vi "S4GUI_002.vi"(7 "Tab ObsEng":enum32{"Obs", "CCD modes", "Eng"}(tab)) -> ()   [LabVIEW 2018] (continued)
            n3730 = call-dynamic "Write Observer.vi"("error in (no error)"=w8546, "Observer"=w8544, "Interface in"=w8548) -> ("error out"=w8545:errorcluster, "Interface out"=w8547:refnum<class "Interface.lvclass">)  [unwired: 7 in]
            n3731 = call-dynamic "Write # Images.vi"("error in (no error)"=w8545, "# Images"="Exp ch4", "Interface in"=w8547) -> ("error out"=w8551:errorcluster, "Interface out"=w8552:refnum<class "Interface.lvclass">)  [unwired: 7 in]
            n3732 = property on="Exposure Time ch4" class="Slide (strict)"("Scale.Maximum"="Exptime ch4", "Scale.Minimum"=0.0 ("Scale.Range:Minimum")) -> ()  [unwired: 2 in, 2 out]
            n3733 = property on="Exposures Done ch4" class="Slide (strict)"("Scale.Maximum"="Exp ch4", "Scale.Minimum"=0.0 ("Scale.Range:Minimum")) -> ()  [unwired: 2 in, 2 out]
            n3734 = call-dynamic "Write Interface.vi"("error in (no error)"=w8551, "Interface.lvclass"=w8552, "Channel in"=w8579) -> ("error out"=w8561:errorcluster, "Channel out"=w8562:refnum<class "Channel.lvclass">)  [unwired: 7 in]
            n3735 = property on="Cycles Done ch4" class="Slide (strict)"("Scale.Maximum"=w8533, "Scale.Minimum"=0.0 ("Scale.Range:Minimum")) -> ()  [unwired: 2 in, 2 out]
            n3736 = call-dynamic "Write ciclos.vi"("error in (no error)"=w8561, "ciclos"=w8533, "Channel in"=w8562) -> ("error out"=w8542:errorcluster, "Channel out"=w8543:refnum<class "Channel.lvclass">)  [unwired: 7 in]
            n3737 = call-dynamic "Write sequencias.vi"("error in (no error)"=w8542, "sequencias"=w8531, "Channel in"=w8543) -> ("error out"=w8541:errorcluster, "Channel out"=w8540:refnum<class "Channel.lvclass">)  [unwired: 7 in]
            n3738 = call-dynamic "Write Channel.vi"("error in (no error)"=w8541, "Channel.lvclass"=w8540, "Acquisition in"=w8568) -> ("error out"=w8508:errorcluster, "Acquisition out"=w8509:refnum<class "Acquisition.lvclass">)  [unwired: 7 in]
            n3739 = call-dynamic "CalcCubeDuration.vi"("error in (no error)"=w8508, "Acquisition in"=w8509) -> ("error out"=w8507:errorcluster, "Acquisition out"=w8506:refnum<class "Acquisition.lvclass">)  [unwired: 8 in]
            n3740 = call-dynamic "Write sequencias.vi"("error in (no error)"=w8507, "sequencias"=w8531, "S4GUI in"=w8514) -> ("error out"=w8537:errorcluster, "S4GUI out"=w8536:refnum<class "S4GUI.lvclass">)  [unwired: 7 in]
            n3741 = call-dynamic "Write ciclos.vi"("error in (no error)"=w8537, "ciclos"=w8533, "S4ACS_GUI in"=w8536) -> ("error out"=w8538:errorcluster, "S4ACS_GUI out"=w8539:refnum<class "S4GUI.lvclass">)  [unwired: 7 in]
            n3742 = call-dynamic "Write TotalCiclos.vi"("error in (no error)"=w8538, "TotalCiclos"=w8533, "S4GUI in"=w8539) -> ("error out"=w8534:errorcluster, "S4GUI out"=w8535:refnum<class "S4GUI.lvclass">)  [unwired: 7 in]
          }
        }
        n3743 = call-dynamic "Write AcquisitionD.vi"("error in (no error)"=w8452, "Acquisition.lvclass"=w8467, "S4ACS_GUI in"=w8451) -> ("error out"=w8466:errorcluster, "S4ACS_GUI out"=w8463:refnum<class "S4GUI.lvclass">)  [unwired: 7 in]
      }
      event "Exptime ch1": Value Change {
        n3744 = event-data() -> ("NewVal"=w8618:dbl)  [unwired: 1 in]
        n3745 = call-dynamic "Read AcquisitionA.vi"("error in (no error)"=w8617, "S4ACS_GUI in"=w8616) -> ("error out"=w8632:errorcluster, "Acquisition.lvclass"=w8633:refnum<class "Acquisition.lvclass">, "S4ACS_GUI out"=w8630:refnum<class "S4GUI.lvclass">)  [unwired: 7 in]
        n3746 = call-dynamic "Read Channel.vi"("error in (no error)"=w8632, "Acquisition in"=w8633) -> ("error out"=w8621:errorcluster, "Channel.lvclass"=w8622:refnum<class "Channel.lvclass">, "Acquisition out"=w8623:refnum<class "Acquisition.lvclass">)  [unwired: 7 in]
        n3747 = call-dynamic "Read Interface.vi"("error in (no error)"=w8621, "Channel in"=w8622) -> ("error out"=w8627:errorcluster, "Interface.lvclass"=w8628:refnum<class "Interface.lvclass">, "Channel out"=w8626:refnum<class "Channel.lvclass">)  [unwired: 7 in]
        n3748 = call "Write Exposure Time.vi"("error in (no error)"=w8627, "Exposure Time"=w8618, "Interface in"=w8628) -> ("error out"=w8619:errorcluster, "Interface out"=w8620:refnum<class "Interface.lvclass">)  [unwired: 7 in]
        n3749 = call-dynamic "Write Interface.vi"("error in (no error)"=w8619, "Interface.lvclass"=w8620, "Channel in"=w8626) -> ("error out"=w8625:errorcluster, "Channel out"=w8624:refnum<class "Channel.lvclass">)  [unwired: 7 in]
        n3750 = call-dynamic "Write Channel.vi"("error in (no error)"=w8625, "Channel.lvclass"=w8624, "Acquisition in"=w8623) -> ("error out"=w8629:errorcluster, "Acquisition out"=w8631:refnum<class "Acquisition.lvclass">)  [unwired: 7 in]
        n3751 = call-dynamic "Write AcquisitionA.vi"("error in (no error)"=w8629, "Acquisition.lvclass"=w8631, "S4ACS_GUI in"=w8630) -> ("error out"=w8615:errorcluster, "S4ACS_GUI out"=w8614:refnum<class "S4GUI.lvclass">)  [unwired: 7 in]
      }
      event "Exptime ch2": Value Change {
        n3752 = event-data() -> ("NewVal"=w8638:dbl)  [unwired: 1 in]
        n3753 = call "Read AcquisitionB.vi"("error in (no error)"=w8637, "S4ACS_GUI in"=w8636) -> ("error out"=w8652:errorcluster, "Acquisition.lvclass"=w8653:refnum<class "Acquisition.lvclass">, "S4ACS_GUI out"=w8650:refnum<class "S4GUI.lvclass">)  [unwired: 7 in]
        n3754 = call-dynamic "Read Channel.vi"("error in (no error)"=w8652, "Acquisition in"=w8653) -> ("error out"=w8641:errorcluster, "Channel.lvclass"=w8642:refnum<class "Channel.lvclass">, "Acquisition out"=w8643:refnum<class "Acquisition.lvclass">)  [unwired: 7 in]
        n3755 = call-dynamic "Read Interface.vi"("error in (no error)"=w8641, "Channel in"=w8642) -> ("error out"=w8647:errorcluster, "Interface.lvclass"=w8648:refnum<class "Interface.lvclass">, "Channel out"=w8646:refnum<class "Channel.lvclass">)  [unwired: 7 in]
        n3756 = call "Write Exposure Time.vi"("error in (no error)"=w8647, "Exposure Time"=w8638, "Interface in"=w8648) -> ("error out"=w8639:errorcluster, "Interface out"=w8640:refnum<class "Interface.lvclass">)  [unwired: 7 in]
        n3757 = call-dynamic "Write Interface.vi"("error in (no error)"=w8639, "Interface.lvclass"=w8640, "Channel in"=w8646) -> ("error out"=w8645:errorcluster, "Channel out"=w8644:refnum<class "Channel.lvclass">)  [unwired: 7 in]
        n3758 = call-dynamic "Write Channel.vi"("error in (no error)"=w8645, "Channel.lvclass"=w8644, "Acquisition in"=w8643) -> ("error out"=w8649:errorcluster, "Acquisition out"=w8651:refnum<class "Acquisition.lvclass">)  [unwired: 7 in]
        n3759 = call "Write AcquisitionB.vi"("error in (no error)"=w8649, "Acquisition.lvclass"=w8651, "S4ACS_GUI in"=w8650) -> ("error out"=w8635:errorcluster, "S4ACS_GUI out"=w8634:refnum<class "S4GUI.lvclass">)  [unwired: 7 in]
      }
      event "Exptime ch3": Value Change {
        n3760 = event-data() -> ("NewVal"=w8658:dbl)  [unwired: 1 in]
        n3761 = call-dynamic "Read AcquisitionC.vi"("error in (no error)"=w8657, "S4ACS_GUI in"=w8656) -> ("error out"=w8672:errorcluster, "Acquisition.lvclass"=w8673:refnum<class "Acquisition.lvclass">, "S4ACS_GUI out"=w8670:refnum<class "S4GUI.lvclass">)  [unwired: 7 in]
        n3762 = call-dynamic "Read Channel.vi"("error in (no error)"=w8672, "Acquisition in"=w8673) -> ("error out"=w8661:errorcluster, "Channel.lvclass"=w8662:refnum<class "Channel.lvclass">, "Acquisition out"=w8663:refnum<class "Acquisition.lvclass">)  [unwired: 7 in]
        n3763 = call-dynamic "Read Interface.vi"("error in (no error)"=w8661, "Channel in"=w8662) -> ("error out"=w8667:errorcluster, "Interface.lvclass"=w8668:refnum<class "Interface.lvclass">, "Channel out"=w8666:refnum<class "Channel.lvclass">)  [unwired: 7 in]
        n3764 = call "Write Exposure Time.vi"("error in (no error)"=w8667, "Exposure Time"=w8658, "Interface in"=w8668) -> ("error out"=w8659:errorcluster, "Interface out"=w8660:refnum<class "Interface.lvclass">)  [unwired: 7 in]
        n3765 = call-dynamic "Write Interface.vi"("error in (no error)"=w8659, "Interface.lvclass"=w8660, "Channel in"=w8666) -> ("error out"=w8665:errorcluster, "Channel out"=w8664:refnum<class "Channel.lvclass">)  [unwired: 7 in]
        n3766 = call-dynamic "Write Channel.vi"("error in (no error)"=w8665, "Channel.lvclass"=w8664, "Acquisition in"=w8663) -> ("error out"=w8669:errorcluster, "Acquisition out"=w8671:refnum<class "Acquisition.lvclass">)  [unwired: 7 in]
        n3767 = call-dynamic "Write AcquisitionC.vi"("error in (no error)"=w8669, "Acquisition.lvclass"=w8671, "S4ACS_GUI in"=w8670) -> ("error out"=w8655:errorcluster, "S4ACS_GUI out"=w8654:refnum<class "S4GUI.lvclass">)  [unwired: 7 in]
      }
      event "Exptime ch4": Value Change {
        n3768 = event-data() -> ("NewVal"=w8678:dbl)  [unwired: 1 in]
        n3769 = call-dynamic "Read AcquisitionD.vi"("error in (no error)"=w8677, "S4ACS_GUI in"=w8676) -> ("error out"=w8692:errorcluster, "Acquisition.lvclass"=w8693:refnum<class "Acquisition.lvclass">, "S4ACS_GUI out"=w8690:refnum<class "S4GUI.lvclass">)  [unwired: 7 in]
        n3770 = call-dynamic "Read Channel.vi"("error in (no error)"=w8692, "Acquisition in"=w8693) -> ("error out"=w8681:errorcluster, "Channel.lvclass"=w8682:refnum<class "Channel.lvclass">, "Acquisition out"=w8683:refnum<class "Acquisition.lvclass">)  [unwired: 7 in]
        n3771 = call-dynamic "Read Interface.vi"("error in (no error)"=w8681, "Channel in"=w8682) -> ("error out"=w8687:errorcluster, "Interface.lvclass"=w8688:refnum<class "Interface.lvclass">, "Channel out"=w8686:refnum<class "Channel.lvclass">)  [unwired: 7 in]
        n3772 = call "Write Exposure Time.vi"("error in (no error)"=w8687, "Exposure Time"=w8678, "Interface in"=w8688) -> ("error out"=w8679:errorcluster, "Interface out"=w8680:refnum<class "Interface.lvclass">)  [unwired: 7 in]
        n3773 = call-dynamic "Write Interface.vi"("error in (no error)"=w8679, "Interface.lvclass"=w8680, "Channel in"=w8686) -> ("error out"=w8685:errorcluster, "Channel out"=w8684:refnum<class "Channel.lvclass">)  [unwired: 7 in]
        n3774 = call-dynamic "Write Channel.vi"("error in (no error)"=w8685, "Channel.lvclass"=w8684, "Acquisition in"=w8683) -> ("error out"=w8689:errorcluster, "Acquisition out"=w8691:refnum<class "Acquisition.lvclass">)  [unwired: 7 in]
        n3775 = call-dynamic "Write AcquisitionD.vi"("error in (no error)"=w8689, "Acquisition.lvclass"=w8691, "S4ACS_GUI in"=w8690) -> ("error out"=w8675:errorcluster, "S4ACS_GUI out"=w8674:refnum<class "S4GUI.lvclass">)  [unwired: 7 in]
      }
      event "Stop ch1": Value Change {
        n3776 = event-data() -> ()  [unwired: 1 in, 6 out]
        n3777 = disable-structure shown="Enabled" {
          disable-tunnel: w8697 -> [w8730 w8758]
          disable-tunnel: w8696 -> [w8728 w8752]
          disable-tunnel: [w8710 w8751] -> w8695
          disable-tunnel: [w8698 w8758] -> w8694
          frame Disabled {
            # "Para movimento \nda lamina retardadora"
            # "Restaura a última sequência de lâminas"
            n3778 = call-dynamic "Read AcquisitionA.vi"("error in (no error)"=w8728, "S4ACS_GUI in"=w8730) -> ("error out"=w8732:errorcluster, "Acquisition.lvclass"=w8731:refnum<class "Acquisition.lvclass">, "S4ACS_GUI out"=w8729:refnum<class "S4GUI.lvclass">)  [unwired: 7 in]
            n3779 = disable-structure shown="Enabled" {
              disable-tunnel: w8732 -> [w8737 w8748]
              disable-tunnel: w8731 -> [w8736 w8749]
              disable-tunnel: [w8734 w8749] -> w8726
              disable-tunnel: [w8733 w8748] -> w8725
              frame Disabled {
                # "Só precisa enviar comando STOP quando\no controle dos ciclos for feito pelo ACS."
                n3780 = call-dynamic "Read Channel.vi"("error in (no error)"=w8737, "Acquisition in"=w8736) -> ("error out"=w8739:errorcluster, "Channel.lvclass"=w8738:refnum<class "Channel.lvclass">, "Acquisition out"=w8745:refnum<class "Acquisition.lvclass">)  [unwired: 7 in]
                n3781 = call-dynamic "Read State Machine.vi"("error in (no error)"=w8739, "Device in"=w8738) -> ("error out"=w8741:errorcluster, "State Machine.lvclass"=w8740:refnum<class "State Machine.lvclass">, "Device out"=w8743:refnum<class "Channel.lvclass">)  [unwired: 7 in]
                n3782 = call "Next State.vi"("error in (no error)"=w8741, "New_State"=u32 70, "State Machine in"=w8740) -> ("error out"=w8744:errorcluster, "State Machine out"=w8742:refnum<class "State Machine.lvclass">)  [unwired: 7 in]
                n3783 = call-dynamic "Write State Machine.vi"("error in (no error)"=w8744, "State Machine.lvclass"=w8742, "Device in"=w8743) -> ("error out"=w8746:errorcluster, "Device out"=w8747:refnum<class "Channel.lvclass">)  [unwired: 7 in]
                n3784 = call-dynamic "Write Channel.vi"("error in (no error)"=w8746, "Channel.lvclass"=w8747, "Acquisition in"=w8745) -> ("error out"=w8733:errorcluster, "Acquisition out"=w8734:refnum<class "Acquisition.lvclass">)  [unwired: 7 in]
              }
              frame Enabled {
                # "Não precisa enviar comando STOP para o ACS\nenquanto o controle dos ciclos for feito pela GUI."
              }
            }
            n3785 = call-dynamic "Write Acq_state.vi"("error in (no error)"=w8725, "Acq_state"=u32 0, "Acquisition in"=w8726) -> ("error out"=w8724:errorcluster, "Acquisition out"=w8723:refnum<class "Acquisition.lvclass">)  [unwired: 7 in]
            n3786 = call-dynamic "Write AcquisitionA.vi"("error in (no error)"=w8724, "Acquisition.lvclass"=w8723, "S4ACS_GUI in"=w8729) -> ("error out"=w8711:errorcluster, "S4ACS_GUI out"=w8709:refnum<class "S4GUI.lvclass">)  [unwired: 7 in]
            n3787 = call "Read Instrument.lvclass.vi"("error in (no error)"=w8711, "S4ACS_GUI in"=w8709) -> ("error out"=w8718:errorcluster, "Instrument.lvclass"=w8721:refnum<class "Instrument.lvclass">, "S4ACS_GUI out"=w8722:refnum<class "S4GUI.lvclass">)  [unwired: 7 in]
            n3788 = call "Read WPROT.vi"("error in (no error)"=w8718, "Instrument in"=w8721) -> ("error out"=w8717:errorcluster, "Opt_Selector.lvclass"=w8719:refnum<class "Opt_Selector.lvclass">, "Instrument out"=w8720:refnum<class "Instrument.lvclass">)  [unwired: 7 in]
            n3789 = call-dynamic "Read sequencia_ant.vi"("error in (no error)"=w8717, "Opt_Selector in"=w8719) -> ("error out"=w8713:errorcluster, "sequencia_ant"=w8712:u16, "Opt_Selector out"=w8714:refnum<class "Opt_Selector.lvclass">)  [unwired: 7 in]
            n3790 = call-dynamic "Write sequencia.vi"("error in (no error)"=w8713, "sequencia"=w8712, "Opt_Selector in"=w8714) -> ("error out"=w8700:errorcluster, "Opt_Selector out"=w8703:refnum<class "Opt_Selector.lvclass">)  [unwired: 7 in]
            n3791 = call-dynamic "Read State Machine.vi"("error in (no error)"=w8700, "Device in"=w8703) -> ("error out"=w8705:errorcluster, "State Machine.lvclass"=w8708:refnum<class "State Machine.lvclass">, "Device out"=w8702:refnum<class "Opt_Selector.lvclass">)  [unwired: 7 in]
            n3792 = call "Next State.vi"("error in (no error)"=w8705, "New_State"=10, "State Machine in"=w8708) -> ("error out"=w8704:errorcluster, "State Machine out"=w8707:refnum<class "State Machine.lvclass">)  [unwired: 7 in]
            n3793 = call-dynamic "Write State Machine.vi"("error in (no error)"=w8704, "State Machine.lvclass"=w8707, "Device in"=w8702) -> ("error out"=w8699:errorcluster, "Device out"=w8701:refnum<class "Opt_Selector.lvclass">)  [unwired: 7 in]
            n3794 = call "Write WPROT.vi"("error in (no error)"=w8699, "Opt_Selector.lvclass"=w8701, "Instrument in"=w8720) -> ("error out"=w8716:errorcluster, "Instrument out"=w8715:refnum<class "Instrument.lvclass">)  [unwired: 7 in]
            n3795 = call "Write Instrument.lvclass.vi"("error in (no error)"=w8716, "Instrument.lvclass"=w8715, "S4ACS_GUI in"=w8722) -> ("error out"=w8710:errorcluster, "S4ACS_GUI out"=w8698:refnum<class "S4GUI.lvclass">)  [unwired: 7 in]
          }
          frame Enabled {
            w8754 = FALSE ("Wait Until Done")
            n3796 = call <vilib>:"Application Directory.vi"() -> ("Application Directory"=w8750:path)
            n3797 = Build Path(base path=w8750, name or relative path="MsgStop1.vi") -> (appended path=w8757:path)
            n3798 = Open VI Reference(vi path=w8757, error in (no error)=w8752) -> (vi reference=w8756:refnum<vi>, error out=w8755:errorcluster)  [unwired: 4 in]
            n3799 = invoke class="VI" method="Run VI"(reference=w8756, error in=w8755, "Wait until done"=w8754, "Auto Dispose Ref"=w8754) -> (error out=w8751:errorcluster)  [unwired: 1 in, 4 out]
          }
        }
      }
      event "Stop ch2": Value Change {
        n3800 = event-data() -> ()  [unwired: 1 in, 6 out]
        n3801 = disable-structure shown="Enabled" {
          disable-tunnel: w8762 -> [w8795 w8816]
          disable-tunnel: w8761 -> [w8793 w8818]
          disable-tunnel: [w8775 w8817] -> w8760
          disable-tunnel: [w8763 w8816] -> w8759
          frame Disabled {
            # "Para movimento \nda lamina retardadora"
            # "Restaura a última sequência de lâminas"
            n3802 = call "Read AcquisitionB.vi"("error in (no error)"=w8793, "S4ACS_GUI in"=w8795) -> ("error out"=w8797:errorcluster, "Acquisition.lvclass"=w8796:refnum<class "Acquisition.lvclass">, "S4ACS_GUI out"=w8794:refnum<class "S4GUI.lvclass">)  [unwired: 7 in]
            n3803 = disable-structure shown="Enabled" {
              disable-tunnel: w8797 -> [w8802 w8813]
              disable-tunnel: w8796 -> [w8801 w8814]
              disable-tunnel: [w8799 w8814] -> w8791
              disable-tunnel: [w8798 w8813] -> w8790
              frame Disabled {
                # "Só precisa enviar comando STOP quando\no controle dos ciclos for feito pelo ACS."
                n3804 = call-dynamic "Read Channel.vi"("error in (no error)"=w8802, "Acquisition in"=w8801) -> ("error out"=w8804:errorcluster, "Channel.lvclass"=w8803:refnum<class "Channel.lvclass">, "Acquisition out"=w8810:refnum<class "Acquisition.lvclass">)  [unwired: 7 in]
                n3805 = call-dynamic "Read State Machine.vi"("error in (no error)"=w8804, "Device in"=w8803) -> ("error out"=w8806:errorcluster, "State Machine.lvclass"=w8805:refnum<class "State Machine.lvclass">, "Device out"=w8808:refnum<class "Channel.lvclass">)  [unwired: 7 in]
                n3806 = call "Next State.vi"("error in (no error)"=w8806, "New_State"=u32 70, "State Machine in"=w8805) -> ("error out"=w8809:errorcluster, "State Machine out"=w8807:refnum<class "State Machine.lvclass">)  [unwired: 7 in]
                n3807 = call-dynamic "Write State Machine.vi"("error in (no error)"=w8809, "State Machine.lvclass"=w8807, "Device in"=w8808) -> ("error out"=w8811:errorcluster, "Device out"=w8812:refnum<class "Channel.lvclass">)  [unwired: 7 in]
                n3808 = call-dynamic "Write Channel.vi"("error in (no error)"=w8811, "Channel.lvclass"=w8812, "Acquisition in"=w8810) -> ("error out"=w8798:errorcluster, "Acquisition out"=w8799:refnum<class "Acquisition.lvclass">)  [unwired: 7 in]
              }
              frame Enabled {
                # "Não precisa enviar comando STOP para o ACS\nenquanto o controle dos ciclos for feito pela GUI."
              }
            }
            n3809 = call-dynamic "Write Acq_state.vi"("error in (no error)"=w8790, "Acq_state"=u32 0, "Acquisition in"=w8791) -> ("error out"=w8789:errorcluster, "Acquisition out"=w8788:refnum<class "Acquisition.lvclass">)  [unwired: 7 in]
            n3810 = call "Write AcquisitionB.vi"("error in (no error)"=w8789, "Acquisition.lvclass"=w8788, "S4ACS_GUI in"=w8794) -> ("error out"=w8776:errorcluster, "S4ACS_GUI out"=w8774:refnum<class "S4GUI.lvclass">)  [unwired: 7 in]
            n3811 = call "Read Instrument.lvclass.vi"("error in (no error)"=w8776, "S4ACS_GUI in"=w8774) -> ("error out"=w8783:errorcluster, "Instrument.lvclass"=w8786:refnum<class "Instrument.lvclass">, "S4ACS_GUI out"=w8787:refnum<class "S4GUI.lvclass">)  [unwired: 7 in]
            n3812 = call "Read WPROT.vi"("error in (no error)"=w8783, "Instrument in"=w8786) -> ("error out"=w8782:errorcluster, "Opt_Selector.lvclass"=w8784:refnum<class "Opt_Selector.lvclass">, "Instrument out"=w8785:refnum<class "Instrument.lvclass">)  [unwired: 7 in]
            n3813 = call-dynamic "Read sequencia_ant.vi"("error in (no error)"=w8782, "Opt_Selector in"=w8784) -> ("error out"=w8778:errorcluster, "sequencia_ant"=w8777:u16, "Opt_Selector out"=w8779:refnum<class "Opt_Selector.lvclass">)  [unwired: 7 in]
            n3814 = call-dynamic "Write sequencia.vi"("error in (no error)"=w8778, "sequencia"=w8777, "Opt_Selector in"=w8779) -> ("error out"=w8765:errorcluster, "Opt_Selector out"=w8768:refnum<class "Opt_Selector.lvclass">)  [unwired: 7 in]
            n3815 = call-dynamic "Read State Machine.vi"("error in (no error)"=w8765, "Device in"=w8768) -> ("error out"=w8770:errorcluster, "State Machine.lvclass"=w8773:refnum<class "State Machine.lvclass">, "Device out"=w8767:refnum<class "Opt_Selector.lvclass">)  [unwired: 7 in]
            n3816 = call "Next State.vi"("error in (no error)"=w8770, "New_State"=10, "State Machine in"=w8773) -> ("error out"=w8769:errorcluster, "State Machine out"=w8772:refnum<class "State Machine.lvclass">)  [unwired: 7 in]
            n3817 = call-dynamic "Write State Machine.vi"("error in (no error)"=w8769, "State Machine.lvclass"=w8772, "Device in"=w8767) -> ("error out"=w8764:errorcluster, "Device out"=w8766:refnum<class "Opt_Selector.lvclass">)  [unwired: 7 in]
            n3818 = call "Write WPROT.vi"("error in (no error)"=w8764, "Opt_Selector.lvclass"=w8766, "Instrument in"=w8785) -> ("error out"=w8781:errorcluster, "Instrument out"=w8780:refnum<class "Instrument.lvclass">)  [unwired: 7 in]
            n3819 = call "Write Instrument.lvclass.vi"("error in (no error)"=w8781, "Instrument.lvclass"=w8780, "S4ACS_GUI in"=w8787) -> ("error out"=w8775:errorcluster, "S4ACS_GUI out"=w8763:refnum<class "S4GUI.lvclass">)  [unwired: 7 in]
          }
          frame Enabled {
            w8820 = FALSE ("Wait Until Done")
            n3820 = call <vilib>:"Application Directory.vi"() -> ("Application Directory"=w8815:path)
            n3821 = Build Path(base path=w8815, name or relative path="MsgStop2.vi") -> (appended path=w8823:path)
            n3822 = Open VI Reference(vi path=w8823, error in (no error)=w8818) -> (vi reference=w8822:refnum<vi>, error out=w8821:errorcluster)  [unwired: 4 in]
            n3823 = invoke class="VI" method="Run VI"(reference=w8822, error in=w8821, "Wait until done"=w8820, "Auto Dispose Ref"=w8820) -> (error out=w8817:errorcluster)  [unwired: 1 in, 4 out]
          }
        }
      }
      event "Stop ch3": Value Change {
        n3824 = event-data() -> ()  [unwired: 1 in, 6 out]
        n3825 = disable-structure shown="Enabled" {
          disable-tunnel: w8827 -> [w8860 w8881]
          disable-tunnel: w8826 -> [w8858 w8883]
          disable-tunnel: [w8840 w8882] -> w8825
          disable-tunnel: [w8828 w8881] -> w8824
          frame Disabled {
            # "Para movimento \nda lamina retardadora"
            # "Restaura a última sequência de lâminas"
            n3826 = call-dynamic "Read AcquisitionC.vi"("error in (no error)"=w8858, "S4ACS_GUI in"=w8860) -> ("error out"=w8862:errorcluster, "Acquisition.lvclass"=w8861:refnum<class "Acquisition.lvclass">, "S4ACS_GUI out"=w8859:refnum<class "S4GUI.lvclass">)  [unwired: 7 in]
            n3827 = disable-structure shown="Enabled" {
              disable-tunnel: w8862 -> [w8867 w8878]
              disable-tunnel: w8861 -> [w8866 w8879]
              disable-tunnel: [w8864 w8879] -> w8856
              disable-tunnel: [w8863 w8878] -> w8855
              frame Disabled {
                # "Só precisa enviar comando STOP quando\no controle dos ciclos for feito pelo ACS."
                n3828 = call-dynamic "Read Channel.vi"("error in (no error)"=w8867, "Acquisition in"=w8866) -> ("error out"=w8869:errorcluster, "Channel.lvclass"=w8868:refnum<class "Channel.lvclass">, "Acquisition out"=w8875:refnum<class "Acquisition.lvclass">)  [unwired: 7 in]
                n3829 = call-dynamic "Read State Machine.vi"("error in (no error)"=w8869, "Device in"=w8868) -> ("error out"=w8871:errorcluster, "State Machine.lvclass"=w8870:refnum<class "State Machine.lvclass">, "Device out"=w8873:refnum<class "Channel.lvclass">)  [unwired: 7 in]
                n3830 = call "Next State.vi"("error in (no error)"=w8871, "New_State"=u32 70, "State Machine in"=w8870) -> ("error out"=w8874:errorcluster, "State Machine out"=w8872:refnum<class "State Machine.lvclass">)  [unwired: 7 in]
                n3831 = call-dynamic "Write State Machine.vi"("error in (no error)"=w8874, "State Machine.lvclass"=w8872, "Device in"=w8873) -> ("error out"=w8876:errorcluster, "Device out"=w8877:refnum<class "Channel.lvclass">)  [unwired: 7 in]
                n3832 = call-dynamic "Write Channel.vi"("error in (no error)"=w8876, "Channel.lvclass"=w8877, "Acquisition in"=w8875) -> ("error out"=w8863:errorcluster, "Acquisition out"=w8864:refnum<class "Acquisition.lvclass">)  [unwired: 7 in]
              }
              frame Enabled {
                # "Não precisa enviar comando STOP para o ACS\nenquanto o controle dos ciclos for feito pela GUI."
              }
            }
            n3833 = call-dynamic "Write Acq_state.vi"("error in (no error)"=w8855, "Acq_state"=u32 0, "Acquisition in"=w8856) -> ("error out"=w8854:errorcluster, "Acquisition out"=w8853:refnum<class "Acquisition.lvclass">)  [unwired: 7 in]
            n3834 = call-dynamic "Write AcquisitionC.vi"("error in (no error)"=w8854, "Acquisition.lvclass"=w8853, "S4ACS_GUI in"=w8859) -> ("error out"=w8841:errorcluster, "S4ACS_GUI out"=w8839:refnum<class "S4GUI.lvclass">)  [unwired: 7 in]
            n3835 = call "Read Instrument.lvclass.vi"("error in (no error)"=w8841, "S4ACS_GUI in"=w8839) -> ("error out"=w8848:errorcluster, "Instrument.lvclass"=w8851:refnum<class "Instrument.lvclass">, "S4ACS_GUI out"=w8852:refnum<class "S4GUI.lvclass">)  [unwired: 7 in]
            n3836 = call "Read WPROT.vi"("error in (no error)"=w8848, "Instrument in"=w8851) -> ("error out"=w8847:errorcluster, "Opt_Selector.lvclass"=w8849:refnum<class "Opt_Selector.lvclass">, "Instrument out"=w8850:refnum<class "Instrument.lvclass">)  [unwired: 7 in]
            n3837 = call-dynamic "Read sequencia_ant.vi"("error in (no error)"=w8847, "Opt_Selector in"=w8849) -> ("error out"=w8843:errorcluster, "sequencia_ant"=w8842:u16, "Opt_Selector out"=w8844:refnum<class "Opt_Selector.lvclass">)  [unwired: 7 in]
            n3838 = call-dynamic "Write sequencia.vi"("error in (no error)"=w8843, "sequencia"=w8842, "Opt_Selector in"=w8844) -> ("error out"=w8830:errorcluster, "Opt_Selector out"=w8833:refnum<class "Opt_Selector.lvclass">)  [unwired: 7 in]
            n3839 = call-dynamic "Read State Machine.vi"("error in (no error)"=w8830, "Device in"=w8833) -> ("error out"=w8835:errorcluster, "State Machine.lvclass"=w8838:refnum<class "State Machine.lvclass">, "Device out"=w8832:refnum<class "Opt_Selector.lvclass">)  [unwired: 7 in]
            n3840 = call "Next State.vi"("error in (no error)"=w8835, "New_State"=10, "State Machine in"=w8838) -> ("error out"=w8834:errorcluster, "State Machine out"=w8837:refnum<class "State Machine.lvclass">)  [unwired: 7 in]
            n3841 = call-dynamic "Write State Machine.vi"("error in (no error)"=w8834, "State Machine.lvclass"=w8837, "Device in"=w8832) -> ("error out"=w8829:errorcluster, "Device out"=w8831:refnum<class "Opt_Selector.lvclass">)  [unwired: 7 in]
            n3842 = call "Write WPROT.vi"("error in (no error)"=w8829, "Opt_Selector.lvclass"=w8831, "Instrument in"=w8850) -> ("error out"=w8846:errorcluster, "Instrument out"=w8845:refnum<class "Instrument.lvclass">)  [unwired: 7 in]
            n3843 = call "Write Instrument.lvclass.vi"("error in (no error)"=w8846, "Instrument.lvclass"=w8845, "S4ACS_GUI in"=w8852) -> ("error out"=w8840:errorcluster, "S4ACS_GUI out"=w8828:refnum<class "S4GUI.lvclass">)  [unwired: 7 in]
          }
          frame Enabled {
            w8885 = FALSE ("Wait Until Done")
            n3844 = call <vilib>:"Application Directory.vi"() -> ("Application Directory"=w8880:path)
            n3845 = Build Path(base path=w8880, name or relative path="MsgStop3.vi") -> (appended path=w8888:path)
            n3846 = Open VI Reference(vi path=w8888, error in (no error)=w8883) -> (vi reference=w8887:refnum<vi>, error out=w8886:errorcluster)  [unwired: 4 in]
            n3847 = invoke class="VI" method="Run VI"(reference=w8887, error in=w8886, "Wait until done"=w8885, "Auto Dispose Ref"=w8885) -> (error out=w8882:errorcluster)  [unwired: 1 in, 4 out]
          }
        }
      }
      event "Stop ch4": Value Change {
        n3848 = event-data() -> ()  [unwired: 1 in, 6 out]
        n3849 = disable-structure shown="Enabled" {
          disable-tunnel: w8892 -> [w8925 w8946]
          disable-tunnel: w8891 -> [w8923 w8948]
          disable-tunnel: [w8905 w8947] -> w8890
          disable-tunnel: [w8893 w8946] -> w8889
          frame Disabled {
            # "Para movimento \nda lamina retardadora"
            # "Restaura a última sequência de lâminas"
            n3850 = call-dynamic "Read AcquisitionD.vi"("error in (no error)"=w8923, "S4ACS_GUI in"=w8925) -> ("error out"=w8927:errorcluster, "Acquisition.lvclass"=w8926:refnum<class "Acquisition.lvclass">, "S4ACS_GUI out"=w8924:refnum<class "S4GUI.lvclass">)  [unwired: 7 in]
            n3851 = disable-structure shown="Enabled" {
              disable-tunnel: w8927 -> [w8932 w8943]
              disable-tunnel: w8926 -> [w8931 w8944]
              disable-tunnel: [w8929 w8944] -> w8921
              disable-tunnel: [w8928 w8943] -> w8920
              frame Disabled {
                # "Só precisa enviar comando STOP quando\no controle dos ciclos for feito pelo ACS."
                n3852 = call-dynamic "Read Channel.vi"("error in (no error)"=w8932, "Acquisition in"=w8931) -> ("error out"=w8934:errorcluster, "Channel.lvclass"=w8933:refnum<class "Channel.lvclass">, "Acquisition out"=w8940:refnum<class "Acquisition.lvclass">)  [unwired: 7 in]
                n3853 = call-dynamic "Read State Machine.vi"("error in (no error)"=w8934, "Device in"=w8933) -> ("error out"=w8936:errorcluster, "State Machine.lvclass"=w8935:refnum<class "State Machine.lvclass">, "Device out"=w8938:refnum<class "Channel.lvclass">)  [unwired: 7 in]
                n3854 = call "Next State.vi"("error in (no error)"=w8936, "New_State"=u32 70, "State Machine in"=w8935) -> ("error out"=w8939:errorcluster, "State Machine out"=w8937:refnum<class "State Machine.lvclass">)  [unwired: 7 in]
                n3855 = call-dynamic "Write State Machine.vi"("error in (no error)"=w8939, "State Machine.lvclass"=w8937, "Device in"=w8938) -> ("error out"=w8941:errorcluster, "Device out"=w8942:refnum<class "Channel.lvclass">)  [unwired: 7 in]
                n3856 = call-dynamic "Write Channel.vi"("error in (no error)"=w8941, "Channel.lvclass"=w8942, "Acquisition in"=w8940) -> ("error out"=w8928:errorcluster, "Acquisition out"=w8929:refnum<class "Acquisition.lvclass">)  [unwired: 7 in]
              }
              frame Enabled {
                # "Não precisa enviar comando STOP para o ACS\nenquanto o controle dos ciclos for feito pela GUI."
              }
            }
            n3857 = call-dynamic "Write Acq_state.vi"("error in (no error)"=w8920, "Acq_state"=u32 0, "Acquisition in"=w8921) -> ("error out"=w8919:errorcluster, "Acquisition out"=w8918:refnum<class "Acquisition.lvclass">)  [unwired: 7 in]
            n3858 = call-dynamic "Write AcquisitionD.vi"("error in (no error)"=w8919, "Acquisition.lvclass"=w8918, "S4ACS_GUI in"=w8924) -> ("error out"=w8906:errorcluster, "S4ACS_GUI out"=w8904:refnum<class "S4GUI.lvclass">)  [unwired: 7 in]
            n3859 = call "Read Instrument.lvclass.vi"("error in (no error)"=w8906, "S4ACS_GUI in"=w8904) -> ("error out"=w8913:errorcluster, "Instrument.lvclass"=w8916:refnum<class "Instrument.lvclass">, "S4ACS_GUI out"=w8917:refnum<class "S4GUI.lvclass">)  [unwired: 7 in]
            n3860 = call "Read WPROT.vi"("error in (no error)"=w8913, "Instrument in"=w8916) -> ("error out"=w8912:errorcluster, "Opt_Selector.lvclass"=w8914:refnum<class "Opt_Selector.lvclass">, "Instrument out"=w8915:refnum<class "Instrument.lvclass">)  [unwired: 7 in]
            n3861 = call-dynamic "Read sequencia_ant.vi"("error in (no error)"=w8912, "Opt_Selector in"=w8914) -> ("error out"=w8908:errorcluster, "sequencia_ant"=w8907:u16, "Opt_Selector out"=w8909:refnum<class "Opt_Selector.lvclass">)  [unwired: 7 in]
            n3862 = call-dynamic "Write sequencia.vi"("error in (no error)"=w8908, "sequencia"=w8907, "Opt_Selector in"=w8909) -> ("error out"=w8895:errorcluster, "Opt_Selector out"=w8898:refnum<class "Opt_Selector.lvclass">)  [unwired: 7 in]
            n3863 = call-dynamic "Read State Machine.vi"("error in (no error)"=w8895, "Device in"=w8898) -> ("error out"=w8900:errorcluster, "State Machine.lvclass"=w8903:refnum<class "State Machine.lvclass">, "Device out"=w8897:refnum<class "Opt_Selector.lvclass">)  [unwired: 7 in]
            n3864 = call "Next State.vi"("error in (no error)"=w8900, "New_State"=10, "State Machine in"=w8903) -> ("error out"=w8899:errorcluster, "State Machine out"=w8902:refnum<class "State Machine.lvclass">)  [unwired: 7 in]
            n3865 = call-dynamic "Write State Machine.vi"("error in (no error)"=w8899, "State Machine.lvclass"=w8902, "Device in"=w8897) -> ("error out"=w8894:errorcluster, "Device out"=w8896:refnum<class "Opt_Selector.lvclass">)  [unwired: 7 in]
            n3866 = call "Write WPROT.vi"("error in (no error)"=w8894, "Opt_Selector.lvclass"=w8896, "Instrument in"=w8915) -> ("error out"=w8911:errorcluster, "Instrument out"=w8910:refnum<class "Instrument.lvclass">)  [unwired: 7 in]
            n3867 = call "Write Instrument.lvclass.vi"("error in (no error)"=w8911, "Instrument.lvclass"=w8910, "S4ACS_GUI in"=w8917) -> ("error out"=w8905:errorcluster, "S4ACS_GUI out"=w8893:refnum<class "S4GUI.lvclass">)  [unwired: 7 in]
          }
          frame Enabled {
            w8950 = FALSE ("Wait Until Done")
            n3868 = call <vilib>:"Application Directory.vi"() -> ("Application Directory"=w8945:path)
            n3869 = Build Path(base path=w8945, name or relative path="MsgStop4.vi") -> (appended path=w8953:path)
            n3870 = Open VI Reference(vi path=w8953, error in (no error)=w8948) -> (vi reference=w8952:refnum<vi>, error out=w8951:errorcluster)  [unwired: 4 in]
            n3871 = invoke class="VI" method="Run VI"(reference=w8952, error in=w8951, "Wait until done"=w8950, "Auto Dispose Ref"=w8950) -> (error out=w8947:errorcluster)  [unwired: 1 in, 4 out]
          }
        }
      }
      event "Pause ch1": Value Change {
        n3872 = event-data() -> ()  [unwired: 1 in, 6 out]
        n3873 = disable-structure shown="Enabled" {
          disable-tunnel: w8957 -> [w8973 w8985]
          disable-tunnel: [w8971 w8983] -> w8956
          disable-tunnel: w8955 -> [w8970 w8984]
          disable-tunnel: [w8958 w8985] -> w8954
          frame Disabled {
            n3874 = call-dynamic "Read AcquisitionA.vi"("error in (no error)"=w8970, "S4ACS_GUI in"=w8973) -> ("error out"=w8965:errorcluster, "Acquisition.lvclass"=w8964:refnum<class "Acquisition.lvclass">, "S4ACS_GUI out"=w8972:refnum<class "S4GUI.lvclass">)  [unwired: 7 in]
            n3875 = call-dynamic "Read Acq_state.vi"("error in (no error)"=w8965, "Acquisition in"=w8964) -> ("error out"=w8967:errorcluster, "Acq_state"=w8968:u32, "Acquisition out"=w8969:refnum<class "Acquisition.lvclass">)  [unwired: 7 in]
            n3876 = call-dynamic "Write Acq_prevstate.vi"("error in (no error)"=w8967, "Acq_prevstate"=w8968, "Acquisition in"=w8969) -> ("error out"=w8962:errorcluster, "Acquisition out"=w8963:refnum<class "Acquisition.lvclass">)  [unwired: 7 in]
            n3877 = call-dynamic "Write Acq_state.vi"("error in (no error)"=w8962, "Acq_state"=u32 400, "Acquisition in"=w8963) -> ("error out"=w8960:errorcluster, "Acquisition out"=w8961:refnum<class "Acquisition.lvclass">)  [unwired: 7 in]
            n3878 = disable-structure shown="Enabled" {
              disable-tunnel: w8960 -> [w8975 w8981]
              disable-tunnel: [w8974 w8981] -> w8959
              frame Disabled {
                n3879 = property on="Start ch1" class="Bool"(error in=w8975, "BoolText.Text"="RESUME" ("Caption.Text")) -> (error out=w8979:errorcluster)  [unwired: 1 in, 1 out]
                n3880 = property on="Pause ch1" class="Bool"(error in=w8979, "DisabledEnum"=T12."Disabled and Grayed Out" ("Disabled")) -> (error out=w8980:errorcluster)  [unwired: 1 in, 1 out]
                n3881 = property on="Start ch1" class="Bool"(error in=w8980, "DisabledEnum"=T12."Enabled" ("Disabled")) -> (error out=w8974:errorcluster)  [unwired: 1 in, 1 out]
              }
              frame Enabled {
              }
            }
            n3882 = call-dynamic "Write AcquisitionA.vi"("error in (no error)"=w8959, "Acquisition.lvclass"=w8961, "S4ACS_GUI in"=w8972) -> ("error out"=w8971:errorcluster, "S4ACS_GUI out"=w8958:refnum<class "S4GUI.lvclass">)  [unwired: 7 in]
          }
          frame Enabled {
            w8987 = FALSE ("Wait Until Done")
            n3883 = call <vilib>:"Application Directory.vi"() -> ("Application Directory"=w8982:path)
            n3884 = Build Path(base path=w8982, name or relative path="MsgPause1.vi") -> (appended path=w8990:path)
            n3885 = Open VI Reference(vi path=w8990, error in (no error)=w8984) -> (vi reference=w8989:refnum<vi>, error out=w8988:errorcluster)  [unwired: 4 in]
            n3886 = invoke class="VI" method="Run VI"(reference=w8989, error in=w8988, "Wait until done"=w8987, "Auto Dispose Ref"=w8987) -> (error out=w8983:errorcluster)  [unwired: 1 in, 4 out]
          }
        }
      }
      event "Pause ch2": Value Change {
        n3887 = event-data() -> ()  [unwired: 1 in, 6 out]
        n3888 = disable-structure shown="Enabled" {
          disable-tunnel: w8994 -> [w9009 w9011]
          disable-tunnel: [w9007 w9012] -> w8993
          disable-tunnel: w8992 -> [w9006 w9013]
          disable-tunnel: [w8996 w9011] -> w8991
          frame Disabled {
            n3889 = call "Read AcquisitionB.vi"("error in (no error)"=w9006, "S4ACS_GUI in"=w9009) -> ("error out"=w9001:errorcluster, "Acquisition.lvclass"=w9000:refnum<class "Acquisition.lvclass">, "S4ACS_GUI out"=w9008:refnum<class "S4GUI.lvclass">)  [unwired: 7 in]
            n3890 = call-dynamic "Read Acq_state.vi"("error in (no error)"=w9001, "Acquisition in"=w9000) -> ("error out"=w9003:errorcluster, "Acq_state"=w9004:u32, "Acquisition out"=w9005:refnum<class "Acquisition.lvclass">)  [unwired: 7 in]
            n3891 = call-dynamic "Write Acq_prevstate.vi"("error in (no error)"=w9003, "Acq_prevstate"=w9004, "Acquisition in"=w9005) -> ("error out"=w8998:errorcluster, "Acquisition out"=w8999:refnum<class "Acquisition.lvclass">)  [unwired: 7 in]
            n3892 = call-dynamic "Write Acq_state.vi"("error in (no error)"=w8998, "Acq_state"=u32 400, "Acquisition in"=w8999) -> ("error out"=w8995:errorcluster, "Acquisition out"=w8997:refnum<class "Acquisition.lvclass">)  [unwired: 7 in]
            n3893 = call "Write AcquisitionB.vi"("error in (no error)"=w8995, "Acquisition.lvclass"=w8997, "S4ACS_GUI in"=w9008) -> ("error out"=w9007:errorcluster, "S4ACS_GUI out"=w8996:refnum<class "S4GUI.lvclass">)  [unwired: 7 in]
          }
          frame Enabled {
            w9015 = FALSE ("Wait Until Done")
            n3894 = call <vilib>:"Application Directory.vi"() -> ("Application Directory"=w9010:path)
            n3895 = Build Path(base path=w9010, name or relative path="MsgPause2.vi") -> (appended path=w9018:path)
            n3896 = Open VI Reference(vi path=w9018, error in (no error)=w9013) -> (vi reference=w9017:refnum<vi>, error out=w9016:errorcluster)  [unwired: 4 in]
            n3897 = invoke class="VI" method="Run VI"(reference=w9017, error in=w9016, "Wait until done"=w9015, "Auto Dispose Ref"=w9015) -> (error out=w9012:errorcluster)  [unwired: 1 in, 4 out]
          }
        }
      }
      event "Pause ch3": Value Change {
        n3898 = event-data() -> ()  [unwired: 1 in, 6 out]
        n3899 = disable-structure shown="Enabled" {
          disable-tunnel: w9022 -> [w9037 w9039]
          disable-tunnel: [w9035 w9040] -> w9021
          disable-tunnel: w9020 -> [w9034 w9041]
          disable-tunnel: [w9024 w9039] -> w9019
          frame Disabled {
            n3900 = call-dynamic "Read AcquisitionC.vi"("error in (no error)"=w9034, "S4ACS_GUI in"=w9037) -> ("error out"=w9029:errorcluster, "Acquisition.lvclass"=w9028:refnum<class "Acquisition.lvclass">, "S4ACS_GUI out"=w9036:refnum<class "S4GUI.lvclass">)  [unwired: 7 in]
            n3901 = call-dynamic "Read Acq_state.vi"("error in (no error)"=w9029, "Acquisition in"=w9028) -> ("error out"=w9031:errorcluster, "Acq_state"=w9032:u32, "Acquisition out"=w9033:refnum<class "Acquisition.lvclass">)  [unwired: 7 in]
            n3902 = call-dynamic "Write Acq_prevstate.vi"("error in (no error)"=w9031, "Acq_prevstate"=w9032, "Acquisition in"=w9033) -> ("error out"=w9026:errorcluster, "Acquisition out"=w9027:refnum<class "Acquisition.lvclass">)  [unwired: 7 in]
            n3903 = call-dynamic "Write Acq_state.vi"("error in (no error)"=w9026, "Acq_state"=u32 400, "Acquisition in"=w9027) -> ("error out"=w9023:errorcluster, "Acquisition out"=w9025:refnum<class "Acquisition.lvclass">)  [unwired: 7 in]
            n3904 = call-dynamic "Write AcquisitionC.vi"("error in (no error)"=w9023, "Acquisition.lvclass"=w9025, "S4ACS_GUI in"=w9036) -> ("error out"=w9035:errorcluster, "S4ACS_GUI out"=w9024:refnum<class "S4GUI.lvclass">)  [unwired: 7 in]
          }
          frame Enabled {
            w9043 = FALSE ("Wait Until Done")
            n3905 = call <vilib>:"Application Directory.vi"() -> ("Application Directory"=w9038:path)
            n3906 = Build Path(base path=w9038, name or relative path="MsgPause3.vi") -> (appended path=w9046:path)
            n3907 = Open VI Reference(vi path=w9046, error in (no error)=w9041) -> (vi reference=w9045:refnum<vi>, error out=w9044:errorcluster)  [unwired: 4 in]
            n3908 = invoke class="VI" method="Run VI"(reference=w9045, error in=w9044, "Wait until done"=w9043, "Auto Dispose Ref"=w9043) -> (error out=w9040:errorcluster)  [unwired: 1 in, 4 out]
          }
        }
      }
      event "Pause ch4": Value Change {
        n3909 = event-data() -> ()  [unwired: 1 in, 6 out]
        n3910 = disable-structure shown="Enabled" {
          disable-tunnel: w9050 -> [w9065 w9074]
          disable-tunnel: [w9063 w9067] -> w9049
          disable-tunnel: w9048 -> [w9062 w9068]
          disable-tunnel: [w9052 w9074] -> w9047
          frame Disabled {
            n3911 = call-dynamic "Read AcquisitionD.vi"("error in (no error)"=w9062, "S4ACS_GUI in"=w9065) -> ("error out"=w9057:errorcluster, "Acquisition.lvclass"=w9056:refnum<class "Acquisition.lvclass">, "S4ACS_GUI out"=w9064:refnum<class "S4GUI.lvclass">)  [unwired: 7 in]
            n3912 = call-dynamic "Read Acq_state.vi"("error in (no error)"=w9057, "Acquisition in"=w9056) -> ("error out"=w9059:errorcluster, "Acq_state"=w9060:u32, "Acquisition out"=w9061:refnum<class "Acquisition.lvclass">)  [unwired: 7 in]
            n3913 = call-dynamic "Write Acq_prevstate.vi"("error in (no error)"=w9059, "Acq_prevstate"=w9060, "Acquisition in"=w9061) -> ("error out"=w9054:errorcluster, "Acquisition out"=w9055:refnum<class "Acquisition.lvclass">)  [unwired: 7 in]
            n3914 = call-dynamic "Write Acq_state.vi"("error in (no error)"=w9054, "Acq_state"=u32 400, "Acquisition in"=w9055) -> ("error out"=w9051:errorcluster, "Acquisition out"=w9053:refnum<class "Acquisition.lvclass">)  [unwired: 7 in]
            n3915 = call-dynamic "Write AcquisitionD.vi"("error in (no error)"=w9051, "Acquisition.lvclass"=w9053, "S4ACS_GUI in"=w9064) -> ("error out"=w9063:errorcluster, "S4ACS_GUI out"=w9052:refnum<class "S4GUI.lvclass">)  [unwired: 7 in]
          }
          frame Enabled {
            w9070 = FALSE ("Wait Until Done")
            n3916 = call <vilib>:"Application Directory.vi"() -> ("Application Directory"=w9066:path)
            n3917 = Build Path(base path=w9066, name or relative path="MsgPause4.vi") -> (appended path=w9073:path)
            n3918 = Open VI Reference(vi path=w9073, error in (no error)=w9068) -> (vi reference=w9072:refnum<vi>, error out=w9071:errorcluster)  [unwired: 4 in]
            n3919 = invoke class="VI" method="Run VI"(reference=w9072, error in=w9071, "Wait until done"=w9070, "Auto Dispose Ref"=w9070) -> (error out=w9067:errorcluster)  [unwired: 1 in, 4 out]
          }
        }
      }
      event "Stop SM": Value Change {
        w9080 = 0.0 ("Scale.Range:Minor Increment")
        n3920 = event-data() -> ()  [unwired: 1 in, 6 out]
        n3921 = call-dynamic "Write User Event.vi"("error in (no error)"=w9078, "User Event"="STOP SM CLICKED", "S4GUI in"=w9079) -> ("error out"=w9076:errorcluster, "S4GUI out"=w9077:refnum<class "S4GUI.lvclass">)  [unwired: 7 in]
        n3922 = disable-structure shown="Enabled" {
          disable-tunnel: w9077 -> [w9117 w9141]
          disable-tunnel: w9076 -> [w9115 w9142]
          disable-tunnel: [w9102 w9140] -> w9082
          disable-tunnel: [w9086 w9141] -> w9081
          frame Disabled {
            # "Não precisa enviar comando STOP para o ACS\nenquanto o controle dos ciclos for feito pela GUI."
            # "Para movimento \nda lamina retardadora"
            # "Restaura a sequencia anterior"
            n3923 = call-dynamic "Read AcquisitionA.vi"("error in (no error)"=w9115, "S4ACS_GUI in"=w9117) -> ("error out"=w9119:errorcluster, "Acquisition.lvclass"=w9118:refnum<class "Acquisition.lvclass">, "S4ACS_GUI out"=w9116:refnum<class "S4GUI.lvclass">)  [unwired: 7 in]
            n3924 = disable-structure shown="Enabled" {
              disable-tunnel: [w9133 w9137] -> w9121
              disable-tunnel: [w9132 w9138] -> w9120
              disable-tunnel: w9119 -> [w9124 w9137]
              disable-tunnel: w9118 -> [w9123 w9138]
              frame Disabled {
                n3925 = call-dynamic "Read Channel.vi"("error in (no error)"=w9124, "Acquisition in"=w9123) -> ("error out"=w9126:errorcluster, "Channel.lvclass"=w9125:refnum<class "Channel.lvclass">, "Acquisition out"=w9134:refnum<class "Acquisition.lvclass">)  [unwired: 7 in]
                n3926 = call-dynamic "Read State Machine.vi"("error in (no error)"=w9126, "Device in"=w9125) -> ("error out"=w9128:errorcluster, "State Machine.lvclass"=w9127:refnum<class "State Machine.lvclass">, "Device out"=w9130:refnum<class "Channel.lvclass">)  [unwired: 7 in]
                n3927 = call "Next State.vi"("error in (no error)"=w9128, "New_State"=u32 70, "State Machine in"=w9127) -> ("error out"=w9131:errorcluster, "State Machine out"=w9129:refnum<class "State Machine.lvclass">)  [unwired: 7 in]
                n3928 = call-dynamic "Write State Machine.vi"("error in (no error)"=w9131, "State Machine.lvclass"=w9129, "Device in"=w9130) -> ("error out"=w9135:errorcluster, "Device out"=w9136:refnum<class "Channel.lvclass">)  [unwired: 7 in]
                n3929 = call-dynamic "Write Channel.vi"("error in (no error)"=w9135, "Channel.lvclass"=w9136, "Acquisition in"=w9134) -> ("error out"=w9133:errorcluster, "Acquisition out"=w9132:refnum<class "Acquisition.lvclass">)  [unwired: 7 in]
              }
              frame Enabled {
              }
            }
            n3930 = call-dynamic "Write AcquisitionA.vi"("error in (no error)"=w9121, "Acquisition.lvclass"=w9120, "S4ACS_GUI in"=w9116) -> ("error out"=w9084:errorcluster, "S4ACS_GUI out"=w9085:refnum<class "S4GUI.lvclass">)  [unwired: 7 in]
            n3931 = call-dynamic "Write Obs_state.vi"("error in (no error)"=w9084, "Obs_state"=u32 0, "S4ACS_GUI in"=w9085) -> ("error out"=w9104:errorcluster, "S4ACS_GUI out"=w9105:refnum<class "S4GUI.lvclass">)  [unwired: 7 in]
            n3932 = call "Read Instrument.lvclass.vi"("error in (no error)"=w9104, "S4ACS_GUI in"=w9105) -> ("error out"=w9113:errorcluster, "Instrument.lvclass"=w9111:refnum<class "Instrument.lvclass">, "S4ACS_GUI out"=w9112:refnum<class "S4GUI.lvclass">)  [unwired: 7 in]
            n3933 = call "Read WPROT.vi"("error in (no error)"=w9113, "Instrument in"=w9111) -> ("error out"=w9098:errorcluster, "Opt_Selector.lvclass"=w9101:refnum<class "Opt_Selector.lvclass">, "Instrument out"=w9110:refnum<class "Instrument.lvclass">)  [unwired: 7 in]
            n3934 = call-dynamic "Read sequencia_ant.vi"("error in (no error)"=w9098, "Opt_Selector in"=w9101) -> ("error out"=w9097:errorcluster, "sequencia_ant"=w9099:u16, "Opt_Selector out"=w9100:refnum<class "Opt_Selector.lvclass">)  [unwired: 7 in]
            n3935 = call-dynamic "Write sequencia.vi"("error in (no error)"=w9097, "sequencia"=w9099, "Opt_Selector in"=w9100) -> ("error out"=w9095:errorcluster, "Opt_Selector out"=w9096:refnum<class "Opt_Selector.lvclass">)  [unwired: 7 in]
            n3936 = call-dynamic "Read State Machine.vi"("error in (no error)"=w9095, "Device in"=w9096) -> ("error out"=w9090:errorcluster, "State Machine.lvclass"=w9093:refnum<class "State Machine.lvclass">, "Device out"=w9094:refnum<class "Opt_Selector.lvclass">)  [unwired: 7 in]
            n3937 = call "Next State.vi"("error in (no error)"=w9090, "New_State"=10, "State Machine in"=w9093) -> ("error out"=w9089:errorcluster, "State Machine out"=w9092:refnum<class "State Machine.lvclass">)  [unwired: 7 in]
            n3938 = call-dynamic "Write State Machine.vi"("error in (no error)"=w9089, "State Machine.lvclass"=w9092, "Device in"=w9094) -> ("error out"=w9088:errorcluster, "Device out"=w9087:refnum<class "Opt_Selector.lvclass">)  [unwired: 7 in]
            n3939 = call "Write WPROT.vi"("error in (no error)"=w9088, "Opt_Selector.lvclass"=w9087, "Instrument in"=w9110) -> ("error out"=w9108:errorcluster, "Instrument out"=w9109:refnum<class "Instrument.lvclass">)  [unwired: 7 in]
            n3940 = call "Write Instrument.lvclass.vi"("error in (no error)"=w9108, "Instrument.lvclass"=w9109, "S4ACS_GUI in"=w9112) -> ("error out"=w9107:errorcluster, "S4ACS_GUI out"=w9106:refnum<class "S4GUI.lvclass">)  [unwired: 7 in]
            n3941 = call-dynamic "Write ciclos.vi"("error in (no error)"=w9107, "ciclos"=u32 0, "S4ACS_GUI in"=w9106) -> ("error out"=w9102:errorcluster, "S4ACS_GUI out"=w9086:refnum<class "S4GUI.lvclass">)  [unwired: 7 in]
          }
          frame Enabled {
            w9144 = FALSE ("Wait Until Done")
            n3942 = call <vilib>:"Application Directory.vi"() -> ("Application Directory"=w9139:path)
            n3943 = Build Path(base path=w9139, name or relative path="MsgStopSync.vi") -> (appended path=w9147:path)
            n3944 = Open VI Reference(vi path=w9147, error in (no error)=w9142) -> (vi reference=w9146:refnum<vi>, error out=w9145:errorcluster)  [unwired: 4 in]
            n3945 = invoke class="VI" method="Run VI"(reference=w9146, error in=w9145, "Wait until done"=w9144, "Auto Dispose Ref"=w9144) -> (error out=w9140:errorcluster)  [unwired: 1 in, 4 out]
          }
        }
        n3946 = property on="#Cycles Done" class="Slide (strict)"(error in=w9082, "Scale.Maximum"=w9080, "Scale.Minimum"=w9080) -> (error out=w9083:errorcluster)  [unwired: 1 in, 1 out]
      }
      event "Abort SM": Value Change {
        w9155 = 0.0 ("Scale.Range:Minor Increment")
        n3947 = event-data() -> ()  [unwired: 1 in, 6 out]
        n3948 = call-dynamic "Write User Event.vi"("error in (no error)"=w9151, "User Event"="ABORT SM CLICKED", "S4GUI in"=w9152) -> ("error out"=w9149:errorcluster, "S4GUI out"=w9150:refnum<class "S4GUI.lvclass">)  [unwired: 7 in]
        n3949 = disable-structure shown="Enabled" {
          disable-tunnel: w9150 -> [w9246 w9270]
          disable-tunnel: w9149 -> [w9244 w9272]
          disable-tunnel: [w9158 w9270] -> w9154
          disable-tunnel: [w9157 w9271] -> w9153
          frame Disabled {
            # "Restaura a sequencia anterior"
            # "Para movimento \nda lamina retardadora"
